vi "Interpolate Transform.vi"(1 "r":dbl, 2 "transform 2":T1, 3 "transform 1":T1) -> (0 "interpolation":T1)   [LabVIEW 2017, in "NI_Kinematics.lvlib"]
uses:
  <vilib>/robotics/Kinematics/NI_Kinematics.lvlib
  <vilib>/Analysis/Matrix/Datatypes/RealMatrix.ctl
  <vilib>/Analysis/baseanly.llb/Dot Product.vi
  <vilib>/Analysis/baseanly.llb/Real Dot Product.vi
  <vilib>/Analysis/baseanly.llb/Outer Product.vi
  <vilib>/Analysis/baseanly.llb/Real Outer Product.vi
  <vilib>/robotics/Kinematics/Create Lie Group Matrix.vi
  <vilib>/Analysis/Matrix/Numeric/Add/Add.vi
  <vilib>/Analysis/Matrix/Numeric/Add/Add - RM,RM.vi
  <vilib>/Analysis/Matrix/Numeric/Multiply/Multiply.vi
  <vilib>/Analysis/Matrix/Numeric/Multiply/Multiply - RM,R.vi
  <vilib>/Analysis/Matrix/Numeric/Multiply/Multiply - R,RM.vi
  <vilib>/robotics/Kinematics/Rotation Matrix to Angle Vector.vi
  <vilib>/Analysis/Matrix/NI_Matrix.lvlib
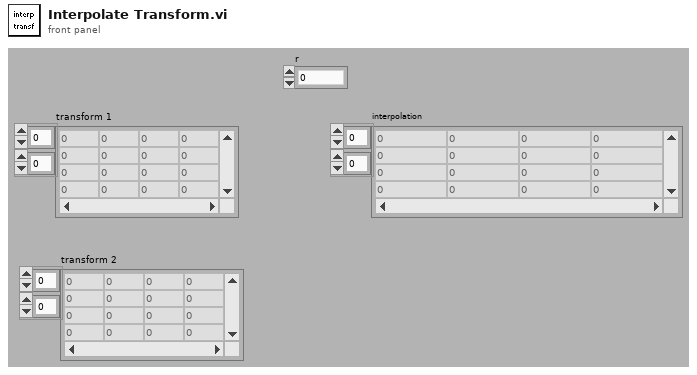
[diagram p1: front panel]
types:
  T1 = typedef "NI_Matrix.lvlib/RealMatrix.ctl" = dbl[][]
  T2 = typedef "NI_Kinematics.lvlib/Quaternion.ctl" = dbl[]
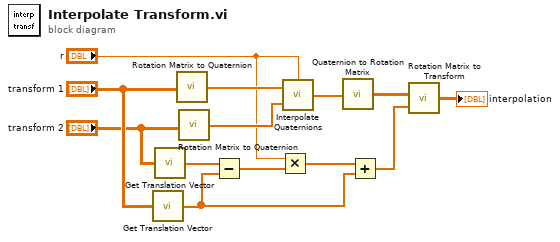
[diagram p0: block diagram]
diagram:
  n1 = call <vilib>:"Get Translation Vector.vi"("transform"="transform 1") -> ("translation vector"=w1:dbl[])
  n2 = call <vilib>:"Get Translation Vector.vi"("transform"="transform 2") -> ("translation vector"=w5:dbl[])
  n3 = call <vilib>:"Rotation Matrix to Quaternion.vi"("rotation matrix"="transform 1") -> ("quaternion"=w13:T2)
  n4 = call <vilib>:"Rotation Matrix to Quaternion.vi"("rotation matrix"="transform 2") -> ("quaternion"=w12:T2)
  n5 = Subtract(x=w5, y=w1) -> (x-y=w6:dbl[])
  n6 = Multiply(x="r", y=w6) -> (x*y=w8:dbl[])
  n7 = call <vilib>:"Interpolate Quaternions.vi"("ratio"="r", "quaternion 2"=w12, "quaternion 1"=w13) -> ("interpolated quaternion"=w11:T2)
  n8 = call <vilib>:"Quaternion to Rotation Matrix.vi"("quaternion"=w11) -> ("rotation matrix"=w10:T1)
  n9 = Add(x=w8, y=w1) -> (x+y=w4:dbl[])
  n10 = call <vilib>:"Rotation Matrix to Transform.vi"("translation vector"=w4, "rotation matrix"=w10) -> ("transform"=→"interpolation":T1)
